vi "SIM Ros solve Wk=F.vi"(2 "F":dbl[](array[numeric]), 3 "Factored W":T1) -> (0 "Error?":bool, 1 "k":dbl[](array[numeric]) format="%.2f")   [LabVIEW 2020]
uses:
  SIM Factored Matrix.ctl
  <resource>/lvanlys.dll
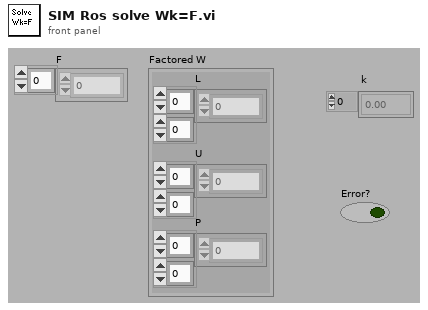
[diagram p1: front panel]
types:
  T1 = typedef "SIM Factored Matrix.ctl" = cluster{"L":dbl[][], "U":dbl[][], "P":i32[][]}
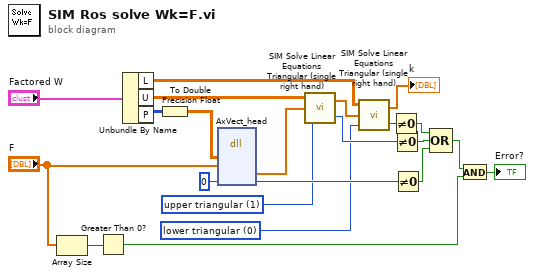
[diagram p0: block diagram]
diagram:
  w1 = 0 items=["lower triangular", "upper triangular", "symmetric matrix"] ("matrix type")
  w2 = 1 items=["lower triangular", "upper triangular", "symmetric matrix"] ("matrix type")
  n1 = Array Size(array="F") -> (size(s)=w18:i32)
  n2 = Greater Than 0?(x=w18) -> (x > 0?=w15:bool)
  n3 = Unbundle By Name("Factored W") -> ("L"=w10:dbl[][], "U"=w14:dbl[][], "P"=w4:i32[][])
  n4 = To Double Precision Float(number=w4) -> (double precision float=w3:dbl[][])
  n5 = dll-call lib="C:/Program Files (x86)/National Instruments/LabVIEW 2020/resource/lvanlys.dll" fn="AxVect_head" label="A x Vector"("A"=w3, "Vector"="F", "output param"=0) -> ("Known Vector"=w6:dbl[], "output param"=w5:i32)  [unwired: 5 in, 4 out]
  n6 = call "SIM Solve Linear Equations Triangular (single right hand).vi"("matrix type"=w2, "Known Vector"=w6, "Input Matrix"=w14) -> ("error"=w13:i32, "Solution Vector"=w9:dbl[])
  n7 = call "SIM Solve Linear Equations Triangular (single right hand).vi"("matrix type"=w1, "Known Vector"=w9, "Input Matrix"=w10) -> ("error"=w12:i32, "Solution Vector"=→"k":dbl[])
  n8 = Not Equal To 0?(x=w12) -> (x != 0?=w19:bool)
  n9 = Not Equal To 0?(x=w13) -> (x != 0?=w20:bool)
  n10 = Not Equal To 0?(x=w5) -> (x != 0?=w21:bool)
  n11 = Compound Arithmetic op=OR(w19, w20, w21) -> (w17:bool)
  n12 = And(x=w17, y=w15) -> (x .and. y?=→"Error?":bool)
